vi "Filter Debug Data.vi"(8 "error in (no error)":errorcluster, 10 "Debug Log":T1[](array[typedef]), 11 "Chronological List In":refnum<class "Chronological List.lvclass">) -> (0 "error out":errorcluster, 2 "Filtered Debug Log":T1[](array[typedef]), 3 "Chronological List Out":refnum<class "Chronological List.lvclass">)   [LabVIEW 2020, in "Chronological List.lvclass"]
uses:
  Chronological List.lvclass
  Debugger/TypeDefs/Debug Data.ctl
  Chronological List.lvclass/Chronological List.ctl
  Debugger/Debugger.lvclass
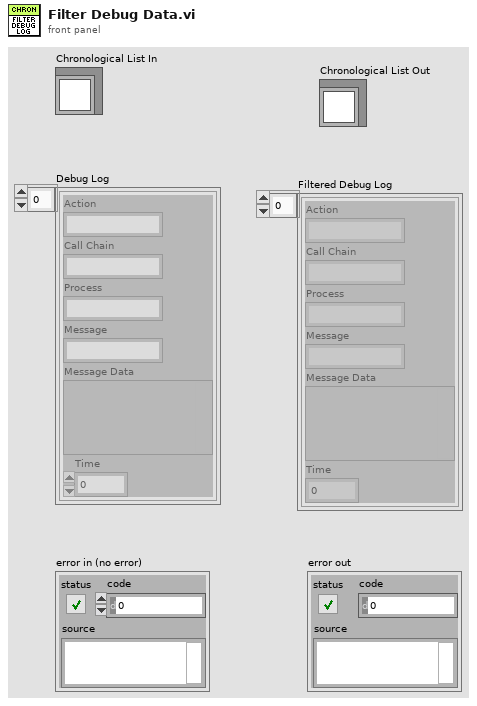
[diagram p1: front panel]
types:
  T1 = typedef "Debugger.lvclass/Debug Data.ctl" = cluster{"Action":string, "Call Chain":string, "Process":string, "Message":string, "Message Data":variant, "Time":u32}
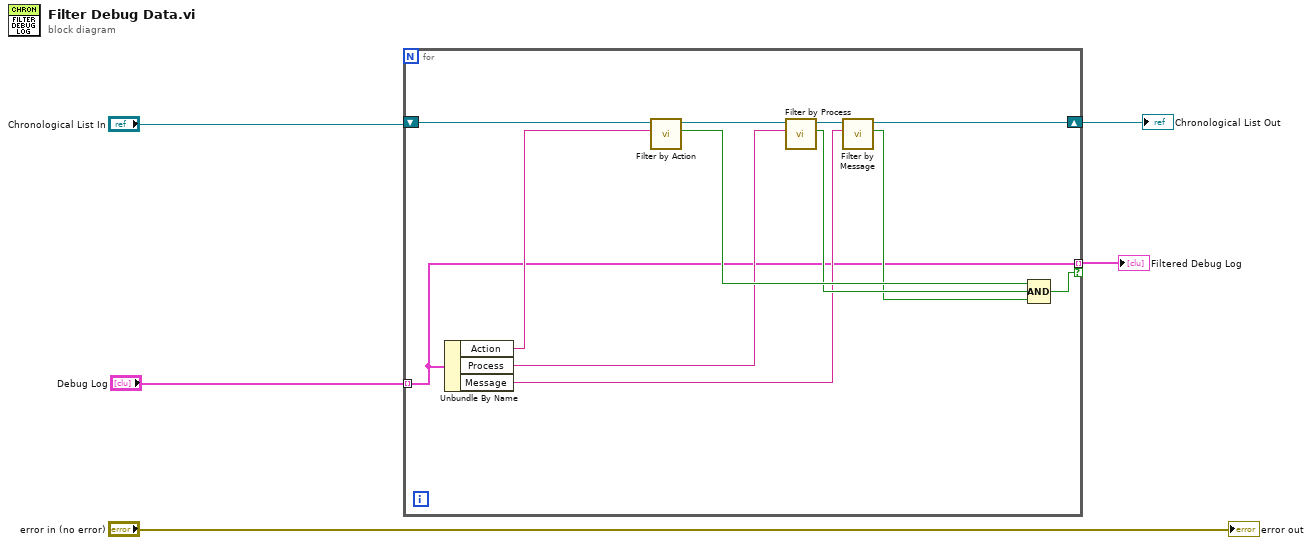
[diagram p0: block diagram]
diagram:
  n1 = for {
    tunnel: "Debug Log" -> [w7] mode=indexing
    shift-right: [w10] -> w2
    shift-left: "Chronological List In" -> [w15]
    tunnel: [w7] -> w1 mode=indexing if=w6
    n2 = Unbundle By Name(w7) -> ("Action"=w17:string, "Process"=w9:string, "Message"=w8:string)
    n3 = call "Filter by Action.vi"("Action"=w17, "Chronological List in"=w15) -> ("Include?"=w16:bool, "Chronological List out"=w12:refnum<class "Chronological List.lvclass">)  [unwired: 8 in]
    n4 = call "Filter by Process.vi"("Process"=w9, "Chronological List in"=w12) -> ("Include?"=w14:bool, "Chronological List out"=w11:refnum<class "Chronological List.lvclass">)  [unwired: 8 in]
    n5 = call "Filter by Message.vi"("Message"=w8, "Chronological List in"=w11) -> ("Include?"=w13:bool, "Chronological List out"=w10:refnum<class "Chronological List.lvclass">)  [unwired: 8 in]
    n6 = Compound Arithmetic op=AND(w16, w14, w13) -> (w6:bool)
  }
  "Chronological List Out" <- w2
  "Filtered Debug Log" <- w1
  "error out" <- "error in (no error)"
